vi "ConfigFile_ErrorBuilder.vi"(5 "KeyNameIn":string, 7 "KeyFound?":bool, 10 "IncomingErrorString":string, 11 "ErrorIn":errorcluster) -> (2 "OutgoingErrorString":string, 3 "ErrorOut":errorcluster)   [LabVIEW 2018]
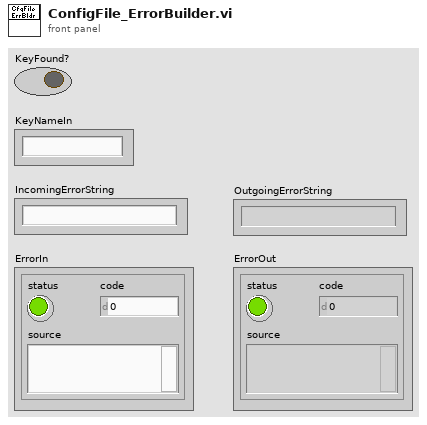
[diagram p1: front panel]
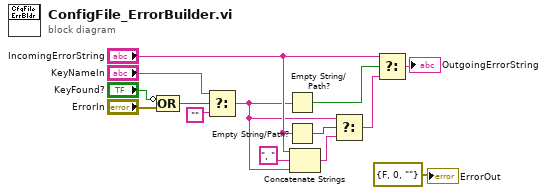
[diagram p0: block diagram]
diagram:
  n1 = Compound Arithmetic op=OR(invert "KeyFound?", "ErrorIn") -> (w12:bool)
  n2 = Select(t="KeyNameIn", s=w12, f="") -> (s? t:f=w1:string)
  n3 = Empty String/Path?(string/path=w1) -> (empty?=w6:bool)
  n4 = Empty String/Path?(string/path="IncomingErrorString") -> (empty?=w13:bool)
  n5 = Concatenate Strings("IncomingErrorString", ", " ("string"), w1) -> (w14:string)
  n6 = Select(t=w1, s=w13, f=w14) -> (s? t:f=w4:string)
  n7 = Select(t="IncomingErrorString", s=w6, f=w4) -> (s? t:f=→"OutgoingErrorString":string)
  "ErrorOut" <- errorcluster {"status"=FALSE, "code"=0, "source"=""} ("ErrorOut")
